vi "Send Control Key Down.vi"(0 "Message Enqueuer in":refnum<class "Message Enqueuer.lvclass">, 1 "ScanCode":i16, 2 "FocusObj":refnum<vi>, 3 "EventFilter Reference":T1, 5 "CtlRef":refnum<vi>, 7 "Time":u32, 9 "Char":i16, 11 "VKey":T3, 12 "Mods":cluster{"Double Click":bool, "Menu Key":bool}, 13 "PlatMods":T2) -> (4 "Filtered EventDataMessage":refnum<class "ControlKeyDownMsg.lvclass">, 15 "error out":errorcluster)   [LabVIEW 2018, in "MVA Framework.lvlib" / "ActorEvents.lvlib" / "ControlKeyDownMsg.lvclass"]
doc: "<License>\nCopyright © 2017 Composed Systems, LLC | All rights reserved\nwww.composed.io\n\nAuthor: Ethan Stern <ethan.stern@composed.io>\n\nThis software is provided \"AS IS\" WITHOUT WARRANTIES, either express or implied, AND IS FOR EDUCATIONAL PURPOSES ONLY.\n</License>"
uses:
  ControlKeyDownMsg.lvclass
  EventDataMessage/EventDataMessage.lvclass
  <vilib>/ActorFramework/Message Enqueuer/Message Enqueuer.lvclass
  <vilib>/event_ctls.llb/eventvkey.ctl
  IEventFilter/IEventFilter.lvclass
  IEventFilter/EventFilter Reference.ctl
panel:
  in  "error in (no error)":errorcluster
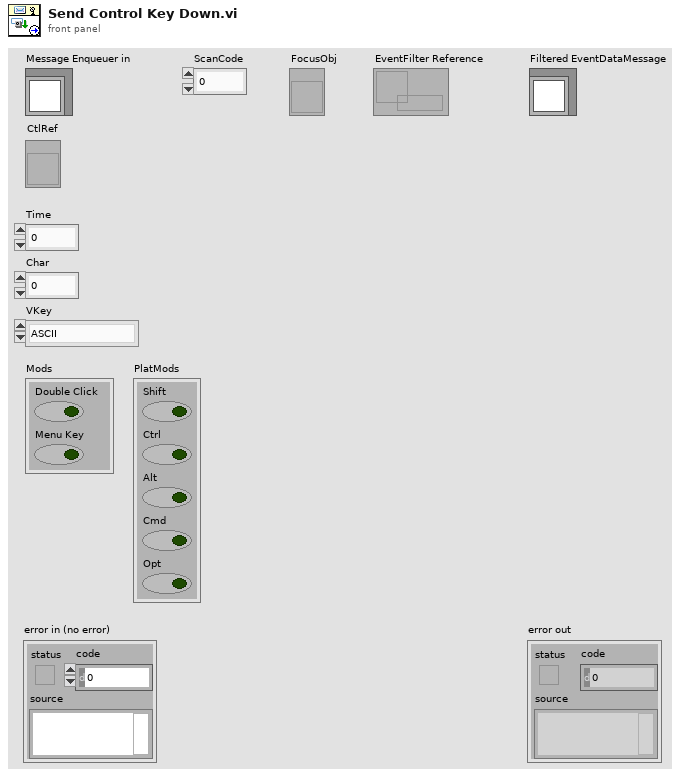
[diagram p1: front panel]
types:
  T1 = typedef "MVA Framework.lvlib/ActorEvents.lvlib/IEventFilter.lvclass/EventFilter Reference.ctl" = refnum<data-value>
  T2 = cluster{"Shift":bool, "Ctrl":bool, "Alt":bool, "Cmd":bool, "Opt":bool}
  T3 = typedef "eventvkey.ctl" = enum16{"ASCII", "Enter", "Return", "Shift", "Ctrl", "Alt", "Cmd", "Opt", "Caps", "NumLock", "Clear", "Break", "Up", "Down", "Left", "Right", "Insert", "Delete", "Home", "End", "PageUp", "PageDown", "Escape", "Help", "Pause", "ScrollLock", "F1", "F2", "F3", "F4", "F5", "F6", "F7", "F8", "F9", "F10", "F11", "F12", "F13", "F14", "F15", "F16", "F17", "F18", "F19", "F20", "F21", "F22", "F23", "F24", "Play", "VolumeUp", "VolumeDown", "Mute", "Two Byte Char"}
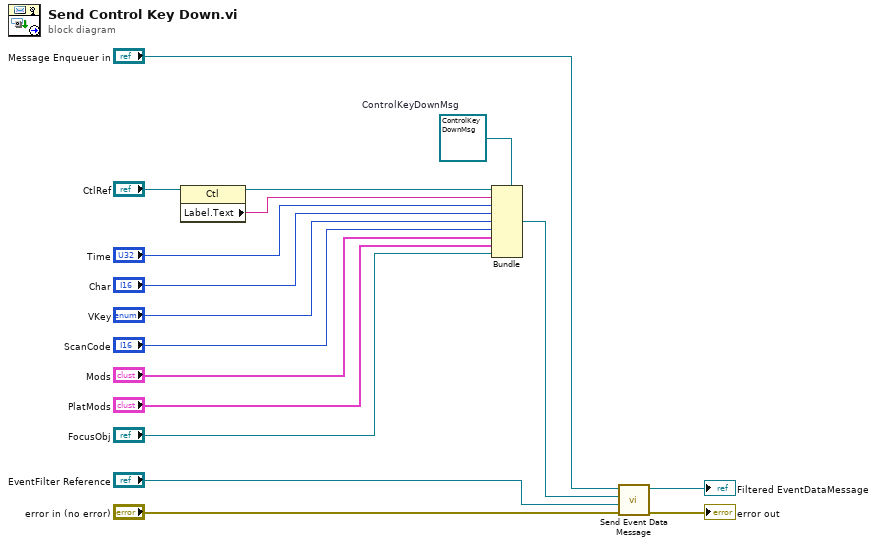
[diagram p0: block diagram]
diagram:
  w17 = refnum<class "ControlKeyDownMsg.lvclass"> refnum  # ControlKeyDownMsg
  n1 = property class="Ctl"(reference="CtlRef") -> (reference out=w11:refnum<vi>, "Label.Text"=w10:string)  [unwired: 1 in, 1 out]
  n2 = Bundle(cluster=w17, w11, w10, "Time", "Char", "VKey", "ScanCode", "Mods", "PlatMods", "FocusObj") -> (w14:refnum<class "ControlKeyDownMsg.lvclass">)
  n3 = call "Send Event Data Message.vi"("error in (no error)"="error in (no error)", "EventFilter Reference"="EventFilter Reference", "EventDataMessage"=w14, "Message Enqueuer in"="Message Enqueuer in") -> ("error out"=→"error out":errorcluster, "Filtered EventDataMessage"=→"Filtered EventDataMessage":refnum<class "ControlKeyDownMsg.lvclass">)  [unwired: 6 in]
